vi "Aliasing Phasor Demo.vi"() -> ()   [LabVIEW 2016]
uses:
  <vilib>/Math Plots/2D Math Plots/2D Compass/2D Compass XCtrl/2D Compass.xctl
  <vilib>/Math Plots/2D Math Plots/2D Compass/2D Compass Datatype/Public/Plot Helper (Vector).vi
  <vilib>/Math Plots/2D Math Plots/2D Compass/2D Compass Datatype/2D Compass Datatype.lvclass
panel:
  out "2D Compass":refnum<class "2D Plot Datatype.lvclass">[](xcontrol)
  in  "Speed":dbl(slide)=8000.0 scale=0.0..10000.0 scale format="%#_6p"
  out "Waveform Chart":waveform(dbl)[](graph)
  in  "Stop":bool
  in  "fs [1/s]":dbl=10.0 format="%#_13g"
  in  "f [Hz]":dbl=1.0 format="%#_13g"
  out "XY Graph":cluster{dbl[], dbl[]}[](graph)
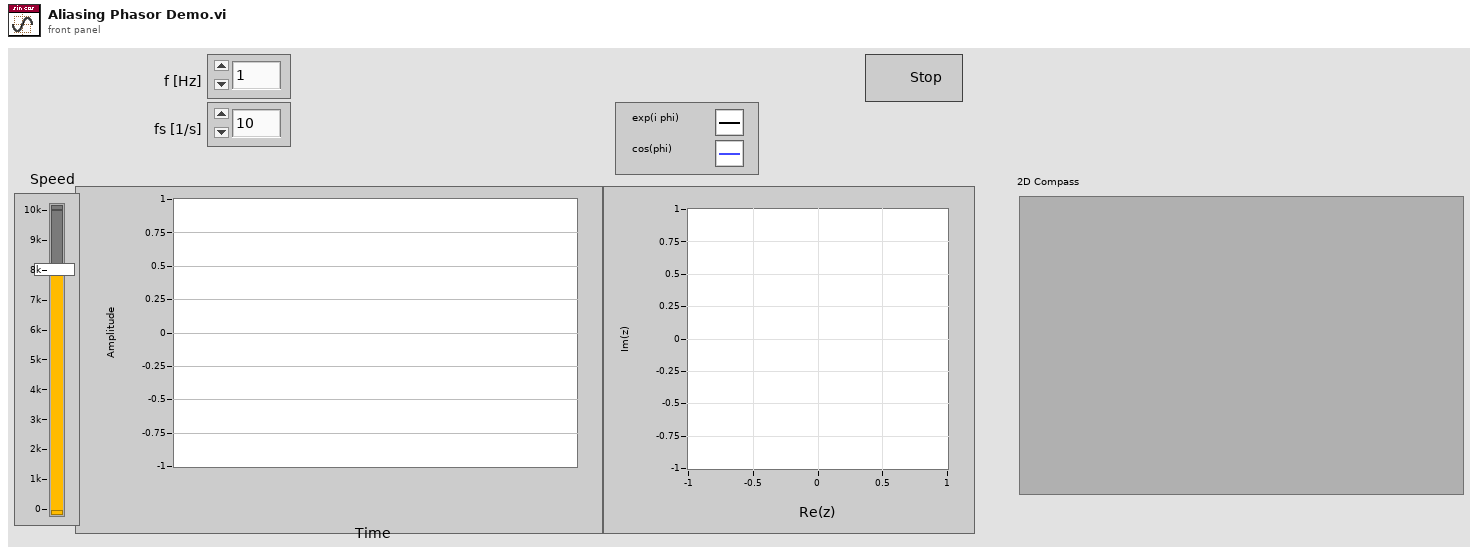
[diagram p1: front panel]
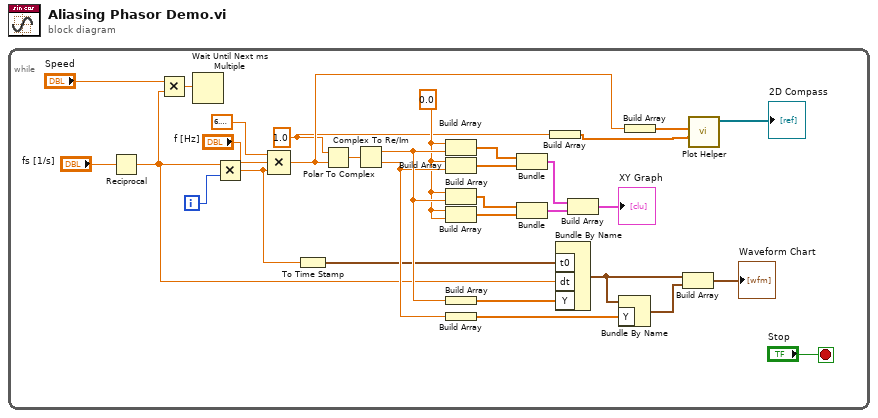
[diagram p0: block diagram]
diagram:
  n1 = while {
    i -> [w26]
    stop <- "Stop" stop-if-true
    w19 = 0.0 ("r")
    w2 = 1.0 ("r")
    n2 = Reciprocal(x="fs [1/s]") -> (1/x=w12:dbl)
    n3 = Multiply(x="Speed", y=w12) -> (x*y=w29:dbl)
    n4 = Wait Until Next ms Multiple(millisecond multiple=w29) -> ()  [unwired: 1 out]
    n5 = Multiply(x=w12, y=w26) -> (x*y=w11:dbl)
    n6 = Compound Arithmetic op=MULTIPLY(6.283185307179586, "f [Hz]", w11) -> (w4:dbl)
    n7 = To Time Stamp(1:w11) -> (0:w10:timestamp)
    n8 = Polar To Complex(1:w4, 2:w2) -> (0:w24:cdb)
    n9 = Complex To Re/Im(x + iy=w24) -> (x=w21:dbl, y=w20:dbl)
    n10 = Build Array(w19, w21) -> (w15:dbl[])
    n11 = Build Array(w19, w20) -> (w14:dbl[])
    n12 = Build Array(w19, w21) -> (w17:dbl[])
    n13 = Build Array(w19, w19) -> (w18:dbl[])
    n14 = Build Array(w21) -> (w5:dbl[])
    n15 = Build Array(w20) -> (w9:dbl[])
    n16 = Bundle(w15, w14) -> (w13:cluster{dbl[], dbl[]})  [unwired: 1 in]
    n17 = Bundle(w17, w18) -> (w16:cluster{dbl[], dbl[]})  [unwired: 1 in]
    n18 = Build Array(w2) -> (w1:dbl[])
    n19 = Bundle By Name("t0"=w10, "dt"=w12, "Y"=w5) -> (w8:waveform(dbl))  [unwired: 1 in]
    n20 = Build Array(w13, w16) -> (→"XY Graph":cluster{dbl[], dbl[]}[])
    n21 = Bundle By Name(cluster=w8, "Y"=w9) -> (w7:waveform(dbl))
    n22 = Build Array(w4) -> (w3:dbl[])
    n23 = Build Array(w8, w7) -> (→"Waveform Chart":waveform(dbl)[])
    n24 = call-poly <vilib>:"Plot Helper.vi"("radius vector"=w1, "theta vector"=w3) -> ("2D Plot Class Obj Array out"=→"2D Compass":refnum<class "2D Plot Datatype.lvclass">[])  [unwired: 2 in, 7 out]
  }
